vi "spectest1.vi"(2 "error in":errorcluster) -> (0 "error out":errorcluster, 1 "LightField Automation out":refnum<class "LightField Automation.lvclass">)   [LabVIEW 2018]
uses:
  C:/ProgramData/Documents/Princeton Instruments/LightField/Add-in and Automation SDK/Samples/LabVIEW Automation/lightfield-automation-labview/LightField Automation.lvclass
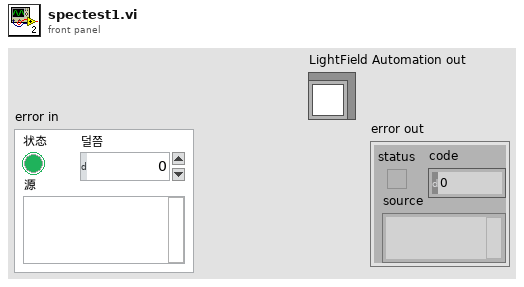
[diagram p1: front panel]
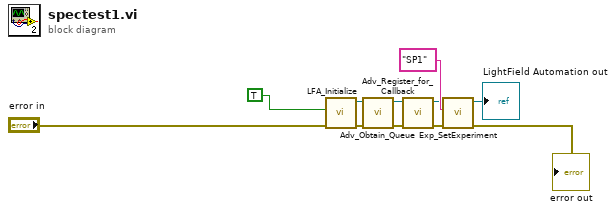
[diagram p0: block diagram]
diagram:
  n1 = call "LFA_Initialize.vi"("error in (no error)"="error in", "Is Visible?"=TRUE) -> ("error out"=w10:errorcluster, "LightField Automation out"=w11:refnum<class "LightField Automation.lvclass">)  [unwired: 8 in]
  n2 = call "Adv_Obtain_Queue.vi"("error in (no error)"=w10, "LightField Automation in"=w11) -> ("error out"=w8:errorcluster, "LightField Automation out"=w9:refnum<class "LightField Automation.lvclass">)  [unwired: 7 in, 1 out]
  n3 = call "Adv_Register_for_Callback.vi"("error in (no error)"=w8, "LightField Automation in"=w9) -> ("error out"=w4:errorcluster, "LightField Automation out"=w5:refnum<class "LightField Automation.lvclass">)  [unwired: 8 in]
  n4 = call "Exp_SetExperiment.vi"("error in (no error)"=w4, "ExperimentName"="SP1" ("Experiment Name"), "LightField Automation in"=w5) -> ("error out"=→"error out":errorcluster, "LightField Automation out"=→"LightField Automation out":refnum<class "LightField Automation.lvclass">)  [unwired: 7 in]
